vi "Exemple_Impute_SimpleImputer.vi"() -> ()   [LabVIEW 2020]
uses:
  Objet/6 - Datasets Transformation/6.4 - Imputation of missing values/SimpleImputer/SimpleImputer.lvclass
panel:
  in  "SimpleImputer":T1={"missing_values"="nan", "strategy"="mean", "fill_value"={"dtype"="None", "str"="None", "int"=0}, "verbose"=0, "copy"=TRUE, "add_indicator"=FALSE}
  out "Data":T2
  out "error out":errorcluster caption="sortie d'erreur"
  in  "y":string[][](array[string])
  in  "X":string[][](array[string])=[["7", "2", "3"], ["4", "nan", "6"], ["10", "5", "9"]]
  in  "error in":errorcluster caption="entrée d'erreur"
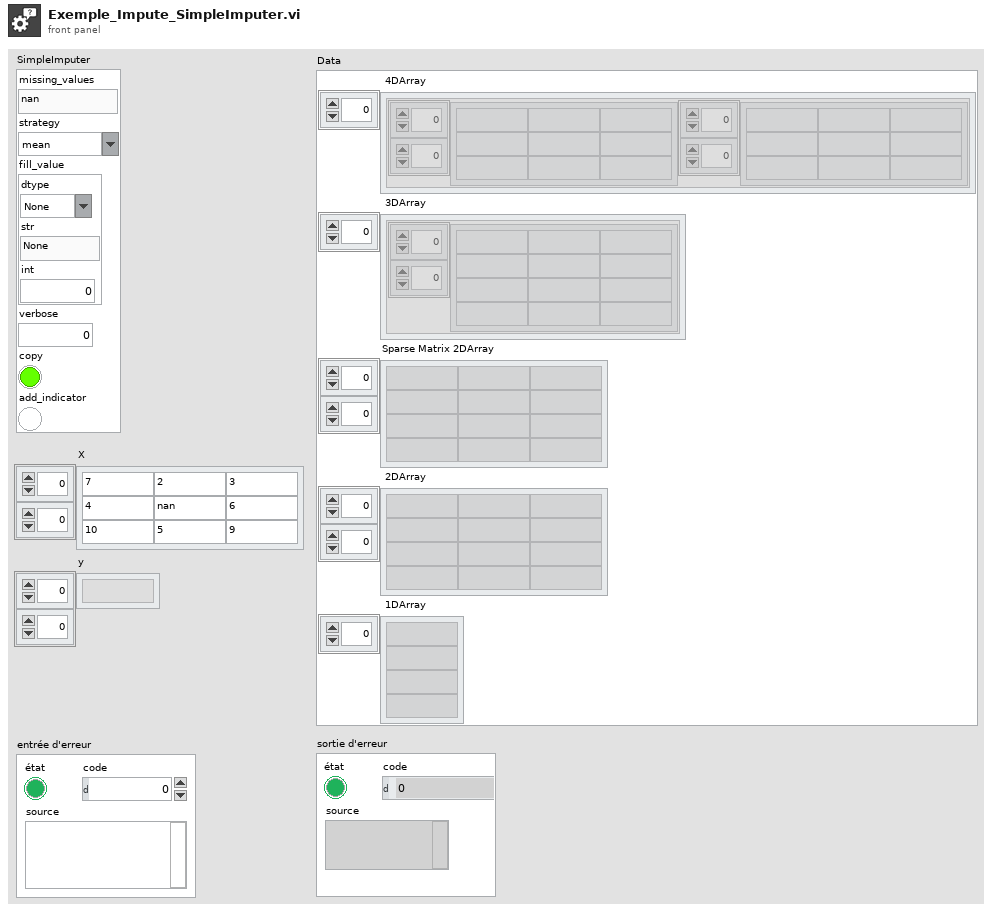
[diagram p1: front panel]
types:
  T1 = cluster{"missing_values":string, "strategy":string, "fill_value":cluster{"dtype":string, "str":string, "int":i32}, "verbose":i32, "copy":bool, "add_indicator":bool}
  T2 = cluster{" 4DArray":cluster{"1":string[][], "2":string[][]}[], " 3DArray":cluster{"Tableau":string[][]}[], "Sparse Matrix 2DArray":string[][], " 2DArray":string[][], " 1DArray":string[]}
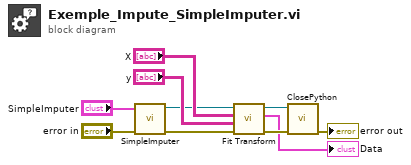
[diagram p0: block diagram]
diagram:
  n1 = call "SimpleImputer.vi"("error in"="error in", "SimpleImputer"="SimpleImputer") -> ("error out"=w7:errorcluster, "SimpleImputer.lvclass"=w6:refnum<class "SimpleImputer.lvclass">)  [unwired: 8 in]
  n2 = call-dynamic "Fit Transform.vi"("error in (no error)"=w7, "y"="y", "X"="X", "SimpleImputer.lvclass"=w6) -> ("error out"=w4:errorcluster, "Data"=→"Data":T2, "SimpleImputer.lvclass"=w5:refnum<class "SimpleImputer.lvclass">)  [unwired: 5 in]
  n3 = call-dynamic "ClosePython.vi"("error in (no error)"=w4, "Scikit-learn en entrée"=w5) -> ("error out"=→"error out":errorcluster)  [unwired: 8 in, 1 out]
